vi "doAction.vi"(8 "error in (no error)":errorcluster, 10 "ContextData":refnum<class "ContextData.lvclass">, 11 "Initialize in":refnum<class "Initialize.lvclass">) -> (0 "error out":errorcluster, 2 "ContextData Out":refnum<class "ContextData.lvclass">, 3 "Initialize out":refnum<class "Initialize.lvclass">)   [LabVIEW 2019, in "Initialize.lvclass"]
uses:
  Initialize.lvclass
  ContextData/ContextData.lvclass
  State/State.lvclass
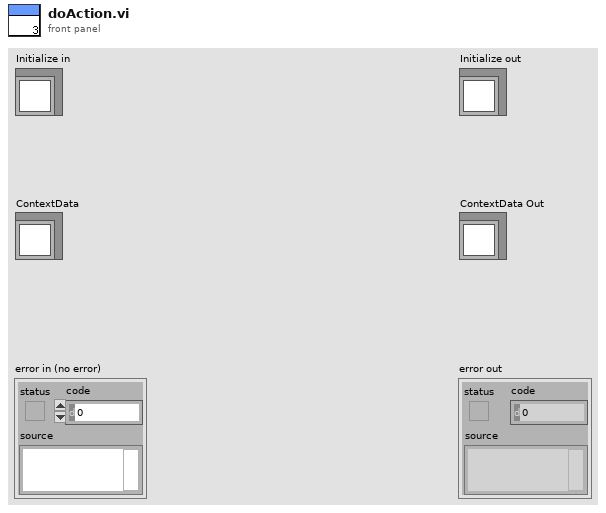
[diagram p1: front panel]
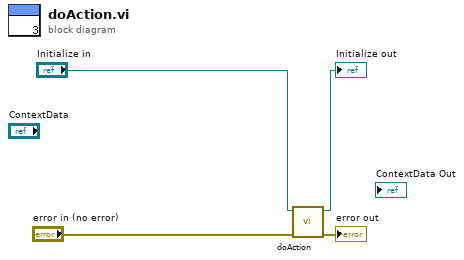
[diagram p0: block diagram]
diagram:
  n1 = call-parent "doAction.vi"("error in (no error)"="error in (no error)", "State in"="Initialize in") -> ("error out"=→"error out":errorcluster, "State out"=→"Initialize out":refnum<class "Initialize.lvclass">)  [unwired: 7 in, 1 out]
